vi "SeCrTs-Drive_Read_A.vi"(8 "error in":errorcluster, 9 "Er":refnum<queue>, 11 "Data FIFO Ref":T1) -> (0 "error out":errorcluster)   [LabVIEW 2022 SP3]
uses:
  RT Support/SeCrTs-RT_Global_R.vi
  RT Controls/SeCrTs-Data FIFO.ctl
panel:
  in  "TCP_Port_Bottom":u16=3000
  in  "TCP_Port_Top":u16=2000
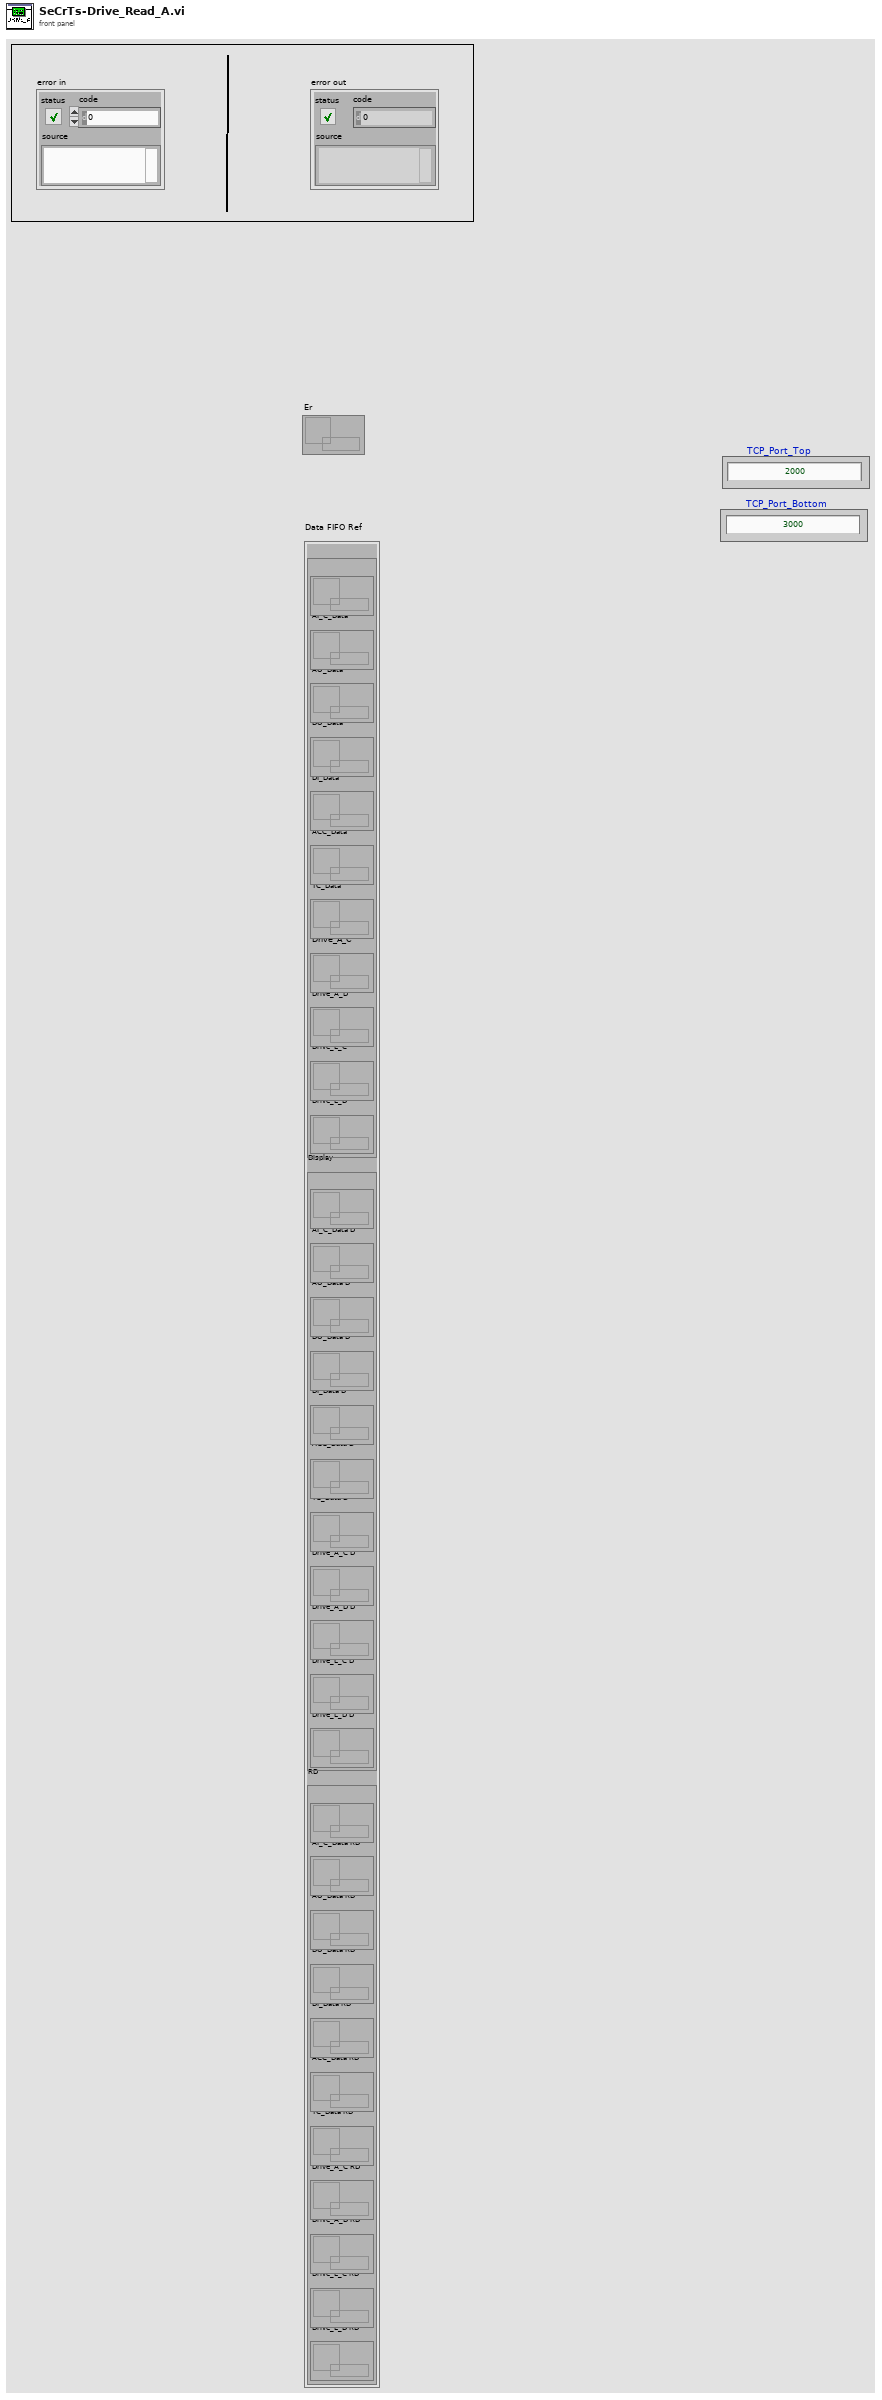
[diagram p1: front panel]
types:
  T1 = typedef "SeCrTs-Data FIFO.ctl" = cluster{"Control":cluster{"AI_V_Data":refnum<queue>, "AI_C_Data":refnum<queue>, "AO_Data":refnum<queue>, "DO_Data":refnum<queue>, "DI_Data":refnum<queue>, "ACC_Data":refnum<queue>, "TC_Data":refnum<queue>, "Drive_A_C":refnum<queue>, "Drive_A_D":refnum<queue>, "Drive_L_C":refnum<queue>, "Drive_L_D":refnum<queue>}, "Display":cluster{"AI_V_Data D":refnum<queue>, "AI_C_Data D":refnum<queue>, "AO_Data D":refnum<queue>, "DO_Data D":refnum<queue>, "DI_Data D":refnum<queue>, "ACC_Data D":refnum<queue>, "TC_Data D":refnum<queue>, "Drive_A_C D":refnum<queue>, "Drive_A_D D":refnum<queue>, "Drive_L_C D":refnum<queue>, "Drive_L_D D":refnum<queue>}, "RD":cluster{"AI_V_Data RD":refnum<queue>, "AI_C_Data RD":refnum<queue>, "AO_Data RD":refnum<queue>, "DO_Data RD":refnum<queue>, "DI_Data RD":refnum<queue>, "ACC_Data RD":refnum<queue>, "TC_Data RD":refnum<queue>, "Drive_A_C RD":refnum<queue>, "Drive_A_D RD":refnum<queue>, "Drive_L_C RD":refnum<queue>, "Drive_L_D RD":refnum<queue>}}
  T2 = enum16{"AI C", "AI V", "AO", "DI", "DO", "TC", "ACC", "DR L", "DR A"}
  T3 = enum16{"Init", "Read 'All'", "Read 'n'", "Read '1'", "Write '1'", "Write 'n'", "Write 'All'"}
  T4 = cluster{"Start DAQ":bool, "Stop DAQ":bool, "RT Stop":bool, "RT Exit":bool, "Start Seq":bool}
  T5 = cluster{"En_Drive_A":bool, "En_Drive_L":bool, "Exit_Drive_A":bool, "Exit_Drive_L":bool}
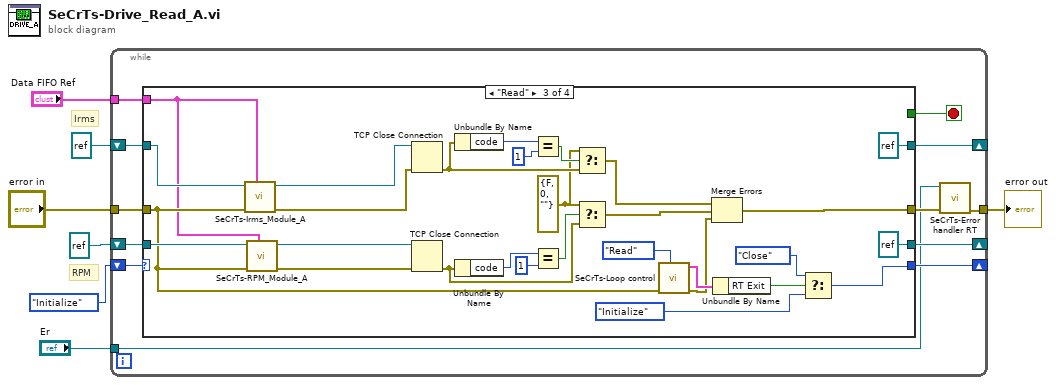
[diagram p0: block diagram]
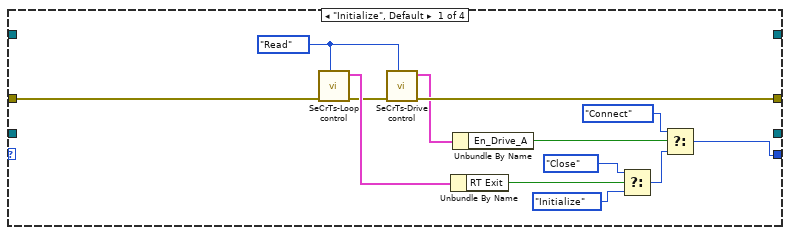
[diagram p2: hidden frame]
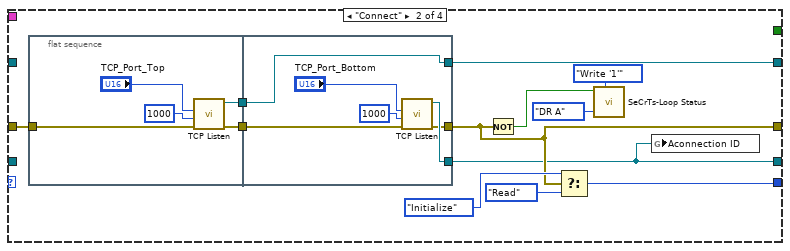
[diagram p3: hidden frame]
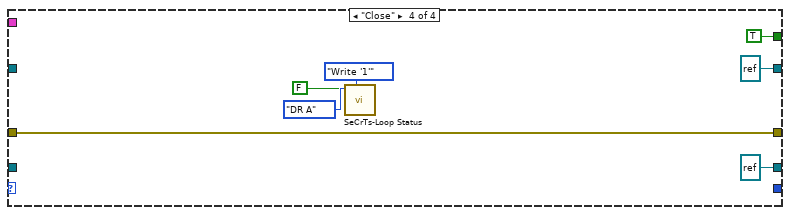
[diagram p4: hidden frame]
diagram:
  # "RPM"
  # "Irms"
  n1 = while {
    shift-right: [w18] -> _
    shift-left: enum16{"Initialize", "Connect", "Read", "Close"}."Initialize" -> [w19]
    tunnel: "error in" -> [w17]
    tunnel: [w9] -> w5
    shift-right: [w16] -> _
    shift-left: refnum<k5> refnum ("connection ID") -> [w14]
    shift-right: [w15] -> _
    shift-left: refnum<k5> refnum ("connection ID") -> [w13]
    tunnel: "Data FIFO Ref" -> [w11]
    tunnel: "Er" -> [w8]
    stop <- w12 stop-if-true
    n2 = case shown="\"Read\"" w19 {
      tunnel: [w32 w38 w82 _] -> w18
      tunnel: w17 -> [w25 w42 w57 w88]
      tunnel: [w24 w37 w70 w88] -> w10
      tunnel: [_ w41 refnum<k5> refnum ("TCP Network Connection out") refnum<k5> refnum ("TCP Network Connection out")] -> w16
      tunnel: [_ w36 refnum<k5> refnum ("TCP Network Connection out") refnum<k5> refnum ("TCP Network Connection out")] -> w15
      tunnel: w14 -> [_ _ w65 _]
      tunnel: w13 -> [_ _ w64 _]
      tunnel: [_ _ _ TRUE] -> w12
      tunnel: w11 -> [_ _ w56 _]
      frame "Initialize", Default {
        w20 = enum16{"Init", "Write", "Read"}."Read" ("Action")
        n3 = call "SeCrTs-Loop control.vi"("Action"=w20, "error in (no error)"=w25) -> ("error Out"=w23:errorcluster, "Loop Control out"=w27:T4)  [unwired: 8 in]
        n4 = call "SeCrTs-Drive control.vi"("Action"=w20, "error in"=w23) -> ("error Out"=w24:errorcluster, "Loop Control Out"=w22:T5)  [unwired: 8 in]
        n5 = Unbundle By Name(w27) -> ("RT Exit"=w26:bool)
        n6 = Unbundle By Name(w22) -> ("En_Drive_A"=w21:bool)
        n7 = Select(t=enum16{"Initialize", "Connect", "Read", "Close"}."Close", s=w26, f=enum16{"Initialize", "Connect", "Read", "Close"}."Initialize") -> (s? t:f=w28:enum16{"Initialize", "Connect", "Read", "Close"})
        n8 = Select(t=enum16{"Initialize", "Connect", "Read", "Close"}."Connect", s=w21, f=w28) -> (s? t:f=w32:enum16{"Initialize", "Connect", "Read", "Close"})
      }
      frame "Connect" {
        n9 = flat-sequence {
          tunnel: w42 -> [w47]
          tunnel: [w46] -> w44
          tunnel: [w45] -> w43
          tunnel: [w55] -> w36
          tunnel: w44 -> [w51]
          tunnel: w43 -> [w54]
          tunnel: [w54] -> w41
          tunnel: [w50] -> w37
          frame #0 {
            n10 = call <vilib>:"TCP Listen.vi"("error in (no error)"=w47, "timeout ms (wait forever: -1)"=1000, "port"="TCP_Port_Top") -> ("error out"=w46:errorcluster, "connection ID"=w45:refnum<k5>)  [unwired: 4 in, 3 out]
          }
          frame #1 {
            n11 = call <vilib>:"TCP Listen.vi"("error in (no error)"=w51, "timeout ms (wait forever: -1)"=1000, "port"="TCP_Port_Bottom") -> ("error out"=w50:errorcluster, "connection ID"=w55:refnum<k5>)  [unwired: 4 in, 3 out]
          }
        }
        n12 = Not(x=w37) -> (.not. x?=w33:bool)
        n13 = Select(t=enum16{"Initialize", "Connect", "Read", "Close"}."Initialize", s=w37, f=enum16{"Initialize", "Connect", "Read", "Close"}."Read") -> (s? t:f=w38:enum16{"Initialize", "Connect", "Read", "Close"})
        n14 = call "SeCrTs-Loop Status.vi"("Option"=T3."Write '1'", "Status"=w33, "Loop"=T2."DR A") -> ()  [unwired: 6 in, 3 out]
        n15 = global write "SeCrTs-RT_Global_R.vi" "Aconnection ID"(w36) -> ()
      }
      frame "Read" {
        w73 = errorcluster {"status"=FALSE, "code"=0, "source"=""} ("error constant")
        n16 = call "SeCrTs-Irms_Module_A.vi"("Data FIFO Ref"=w56, "error in"=w57, "TCP Network Connection in"=w65) -> ("error out"=w66:errorcluster, "TCP Network Connection out"=w67:refnum<k5>)  [unwired: 7 in]
        n17 = call "SeCrTs-RPM_Module_A.vi"("Data FIFO Ref"=w56, "error in (no error)"=w57, "TCP Network Connection in"=w64) -> ("error out"=w62:errorcluster, "TCP Network Connection out"=w63:refnum<k5>)  [unwired: 7 in]
        n18 = TCP Close Connection(connection ID=w67, error in (no error)=w66) -> (error out=w77:errorcluster)  [unwired: 1 in, 1 out]
        n19 = TCP Close Connection(connection ID=w63, error in (no error)=w62) -> (error out=w76:errorcluster)  [unwired: 1 in, 1 out]
        n20 = Unbundle By Name(w77) -> ("code"=w81:i32)
        n21 = Unbundle By Name(w76) -> ("code"=w80:i32)
        n22 = Equal?(x=w81, y=1) -> (x = y?=w78:bool)
        n23 = Equal?(x=w80, y=1) -> (x = y?=w79:bool)
        n24 = Select(t=w73, s=w78, f=w77) -> (s? t:f=w75:errorcluster)
        n25 = Select(t=w73, s=w79, f=w76) -> (s? t:f=w74:errorcluster)
        n26 = call "SeCrTs-Loop control.vi"("Action"=enum16{"Init", "Write", "Read"}."Read", "error in (no error)"=w57) -> ("error Out"=w58:errorcluster, "Loop Control out"=w61:T4)  [unwired: 8 in]
        n27 = Merge Errors(w75, w74, w58) -> (w70:errorcluster)
        n28 = Unbundle By Name(w61) -> ("RT Exit"=w60:bool)
        n29 = Select(t=enum16{"Initialize", "Connect", "Read", "Close"}."Close", s=w60, f=enum16{"Initialize", "Connect", "Read", "Close"}."Initialize") -> (s? t:f=w82:enum16{"Initialize", "Connect", "Read", "Close"})
      }
      frame "Close" {
        n30 = call "SeCrTs-Loop Status.vi"("Option"=T3."Write '1'", "Status"=FALSE, "Loop"=T2."DR A") -> ()  [unwired: 6 in, 3 out]
      }
    }
    n31 = call "SeCrTs-Error handler RT.vi"("error in"=w10, "Message Queue"=w8) -> ("error out"=w9:errorcluster)  [unwired: 8 in, 1 out]
  }
  "error out" <- w5
